vi "Chapter 3.vi"() -> ()   [LabVIEW 2018]
uses:
  <vilib>/Utility/cursorutil.llb/Set Cursor (Icon Pict).vi
panel:
  in  "icon":u16(ring) caption="아이콘"
  in  "정지 버튼":bool
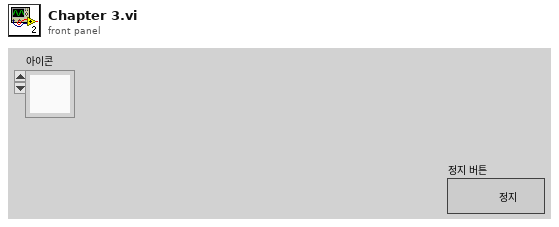
[diagram p1: front panel]
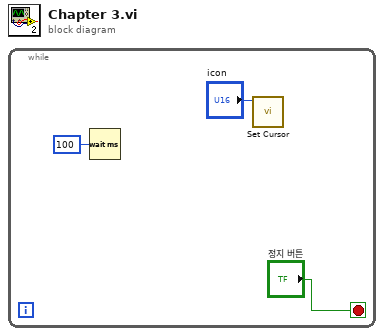
[diagram p0: block diagram]
diagram:
  n1 = while {
    stop <- "정지 버튼" stop-if-true
    n2 = Wait (ms)(milliseconds to wait=u32 100 ("대기 시간 (ms)")) -> ()  [unwired: 1 out]
    n3 = call-poly <vilib>:"Set Cursor.vi"("icon"="icon") -> ()  [unwired: 9 in, 2 out]
  }
